vi "Write Config.vi"(8 "error in (no error)":errorcluster, 10 "Config":T1, 11 "Path":path) -> (0 "error out":errorcluster)   [LabVIEW 2023, in "VI Properties Editor.lvlib"]
doc: "Writes to a config file located at <B>Path</B>."
uses:
  VI Properties Editor.lvlib
  CTLs/Config.ctl
  <vilib>/Utility/config.llb/Write Key (String).vi
  <vilib>/Utility/config.llb/Write Key (Boolean).vi
  <vilib>/Utility/config.llb/NI_LVConfig.lvlib
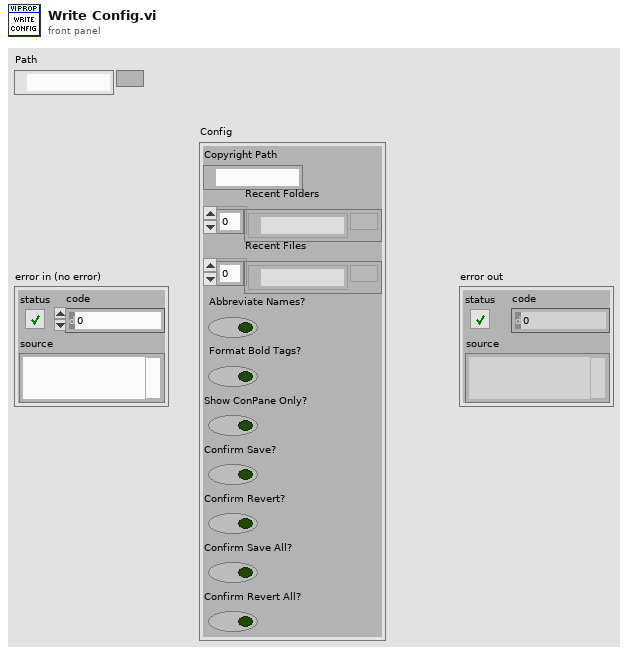
[diagram p1: front panel]
types:
  T1 = typedef "VI Properties Editor.lvlib/Config.ctl" = cluster{"Copyright Path":path, "Recent Folders":path[], "Recent Files":path[], "Abbreviate Names?":bool, "Format Bold Tags?":bool, "Show ConPane Only?":bool, "Confirm Save?":bool, "Confirm Revert?":bool, "Confirm Save All?":bool, "Confirm Revert All?":bool}
  T2 = typedef "NI_LVConfig.lvlib/Config Data RefNum.ctl" = refnum<k1>
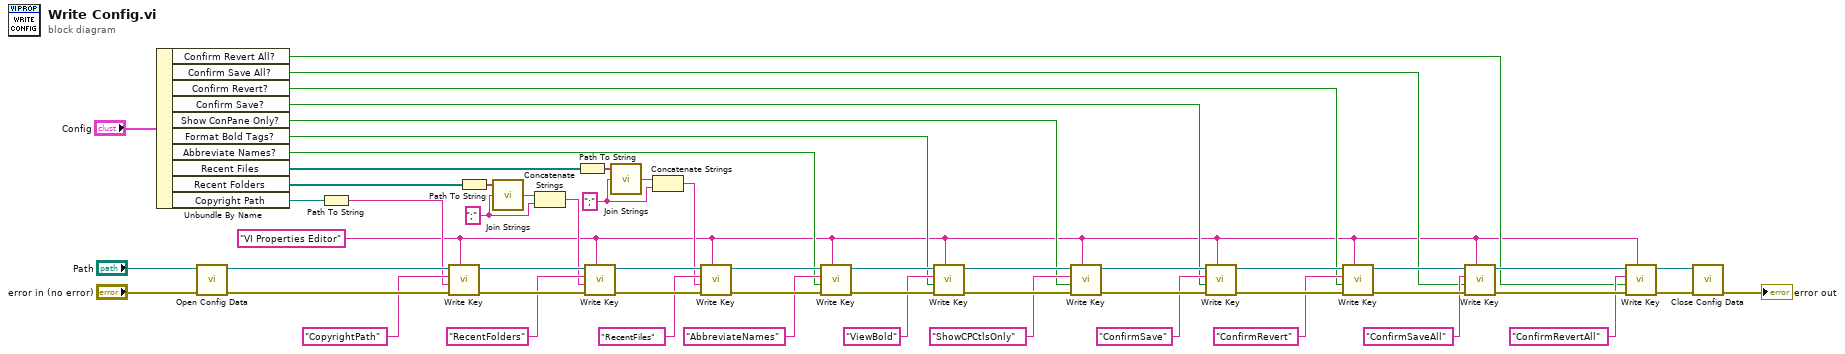
[diagram p0: block diagram]
diagram:
  w19 = ";" ("Separator (,)")
  w21 = ";" ("Separator (,)")
  w3 = "VI Properties Editor" ("section")
  n1 = Unbundle By Name("Config") -> ("Confirm Revert All?"=w4:bool, "Confirm Save All?"=w5:bool, "Confirm Revert?"=w6:bool, "Confirm Save?"=w7:bool, "Show ConPane Only?"=w16:bool, "Format Bold Tags?"=w35:bool, "Abbreviate Names?"=w36:bool, "Recent Files"=w25:path[], "Recent Folders"=w28:path[], "Copyright Path"=w37:path)
  n2 = call <vilib>:"Open Config Data.vi"("error in (no error)"="error in (no error)", "configuration file path"="Path") -> ("error out"=w55:errorcluster, "refnum"=w42:T2)  [unwired: 7 in, 1 out]
  n3 = Path To String(path=w37) -> (string=w33:string)
  n4 = call-poly <vilib>:"Write Key.vi"("section"=w3, "error in (no error)"=w55, "value"=w33, "key"="CopyrightPath", "refnum"=w42) -> ("error out"=w51:errorcluster, "refnum out"=w29:T2)  [unwired: 4 in, 1 out]
  n5 = Path To String(path=w28) -> (string=w27:string[])
  n6 = call <vilib>:"Join Strings.vi"("Separator (,)"=w21, "Strings In"=w27) -> ("String"=w23:string)  [unwired: 1 in]
  n7 = Concatenate Strings(w23, w21) -> (w22:string)
  n8 = Path To String(path=w25) -> (string=w26:string[])
  n9 = call-poly <vilib>:"Write Key.vi"("section"=w3, "error in (no error)"=w51, "value"=w22, "key"="RecentFolders", "refnum"=w29) -> ("error out"=w50:errorcluster, "refnum out"=w30:T2)  [unwired: 4 in, 1 out]
  n10 = call <vilib>:"Join Strings.vi"("Separator (,)"=w19, "Strings In"=w26) -> ("String"=w24:string)  [unwired: 1 in]
  n11 = Concatenate Strings(w24, w19) -> (w20:string)
  n12 = call-poly <vilib>:"Write Key.vi"("section"=w3, "error in (no error)"=w50, "value"=w20, "key"="RecentFiles", "refnum"=w30) -> ("error out"=w49:errorcluster, "refnum out"=w44:T2)  [unwired: 4 in, 1 out]
  n13 = call-poly <vilib>:"Write Key.vi"("section"=w3, "error in (no error)"=w49, "value"=w36, "key"="AbbreviateNames", "refnum"=w44) -> ("error out"=w52:errorcluster, "refnum out"=w39:T2)  [unwired: 4 in, 1 out]
  n14 = call-poly <vilib>:"Write Key.vi"("section"=w3, "error in (no error)"=w52, "value"=w35, "key"="ViewBold", "refnum"=w39) -> ("error out"=w54:errorcluster, "refnum out"=w18:T2)  [unwired: 4 in, 1 out]
  n15 = call-poly <vilib>:"Write Key.vi"("section"=w3, "error in (no error)"=w54, "value"=w16, "key"="ShowCPCtlsOnly", "refnum"=w18) -> ("error out"=w46:errorcluster, "refnum out"=w11:T2)  [unwired: 4 in, 1 out]
  n16 = call-poly <vilib>:"Write Key.vi"("section"=w3, "error in (no error)"=w46, "value"=w7, "key"="ConfirmSave", "refnum"=w11) -> ("error out"=w48:errorcluster, "refnum out"=w10:T2)  [unwired: 4 in, 1 out]
  n17 = call-poly <vilib>:"Write Key.vi"("section"=w3, "error in (no error)"=w48, "value"=w6, "key"="ConfirmRevert", "refnum"=w10) -> ("error out"=w45:errorcluster, "refnum out"=w9:T2)  [unwired: 4 in, 1 out]
  n18 = call-poly <vilib>:"Write Key.vi"("section"=w3, "error in (no error)"=w45, "value"=w5, "key"="ConfirmSaveAll", "refnum"=w9) -> ("error out"=w47:errorcluster, "refnum out"=w8:T2)  [unwired: 4 in, 1 out]
  n19 = call-poly <vilib>:"Write Key.vi"("section"=w3, "error in (no error)"=w47, "value"=w4, "key"="ConfirmRevertAll", "refnum"=w8) -> ("error out"=w2:errorcluster, "refnum out"=w1:T2)  [unwired: 4 in, 1 out]
  n20 = call <vilib>:"Close Config Data.vi"("error in (no error)"=w2, "refnum"=w1) -> ("error out"=→"error out":errorcluster)  [unwired: 8 in, 1 out]
